vi "Linear Ramp [I32].vi"(0 "Increment (1)":i32=1, 3 "# Elements":i32, 4 "Start (0)":i32) -> (5 "Ramp":i32[](array[numeric]))   [LabVIEW 2019]
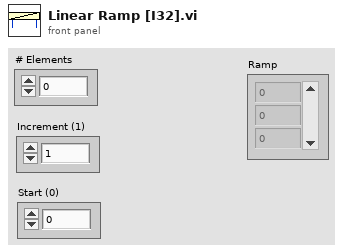
[diagram p1: front panel]
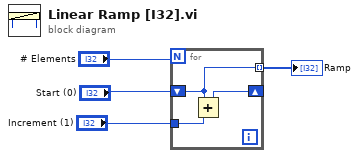
[diagram p0: block diagram]
diagram:
  n1 = for {
    N: "# Elements" -> [_]
    shift-right: [w6] -> _
    shift-left: "Start (0)" -> [w5]
    tunnel: "Increment (1)" -> [w7]
    tunnel: [w5] -> w1 mode=indexing
    n2 = Add(x=w5, y=w7) -> (x+y=w6:i32)
  }
  "Ramp" <- w1
